vi "Loop_SOL.vi"() -> ()   [LabVIEW 2017, in "Wing.lvlib"]
uses:
  Wing.lvlib
  <vilib>/Rock Robotics/WPI/Solenoid/WPI_SolenoidValue.ctl
  <vilib>/Rock Robotics/WPI/Solenoid/WPI_SolenoidChannel.ctl
  <vilib>/Rock Robotics/WPI/Solenoid/WPI_SolenoidOpenSingle.vi
  _SHARE ALL/Global Share All/Global_STOP.vi
  Global_SM Write_Data Out.vi
  <vilib>/Rock Robotics/WPI/Solenoid/WPI_SolenoidSetEnum.vi
  <vilib>/Rock Robotics/WPI/Solenoid/WPI_SolenoidGetEnum.vi
  Global_ACT Write_Data Out.vi
panel:
  out "Value":T1
  out "Solenoid On.Off":bool
  out "Cycle Time (S)":dbl format="%.3g"
  in  "Target Time(ms)":u32=50
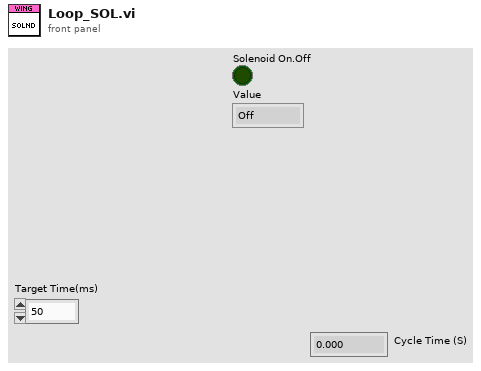
[diagram p1: front panel]
types:
  T1 = typedef "WPI_SolenoidValue.ctl" = enum16{"Off", "On", "Forward", "Reverse"}
  T2 = typedef "WPI_SolenoidChannel.ctl" = enum8{"Solenoid 0", "Solenoid 1", "Solenoid 2", "Solenoid 3", "Solenoid 4", "Solenoid 5", "Solenoid 6", "Solenoid 7", "Invalid"}
  T3 = typedef "WPI_SolenoidDevRef.ctl" = cluster{"DevStatus":errorcluster, "Pneumatics Control Module":u8, "Forward Solenoid Channel":T2, "Reverse Solenoid Channel":T2}
  T4 = cluster{"SolenoidDevRef":T3, "Target Time(ms)":u32, "Current Time":timestamp, "Previous Time":timestamp, "Cycle Time (S)":dbl, "Solenoid On.Off":bool, "Value":T1}
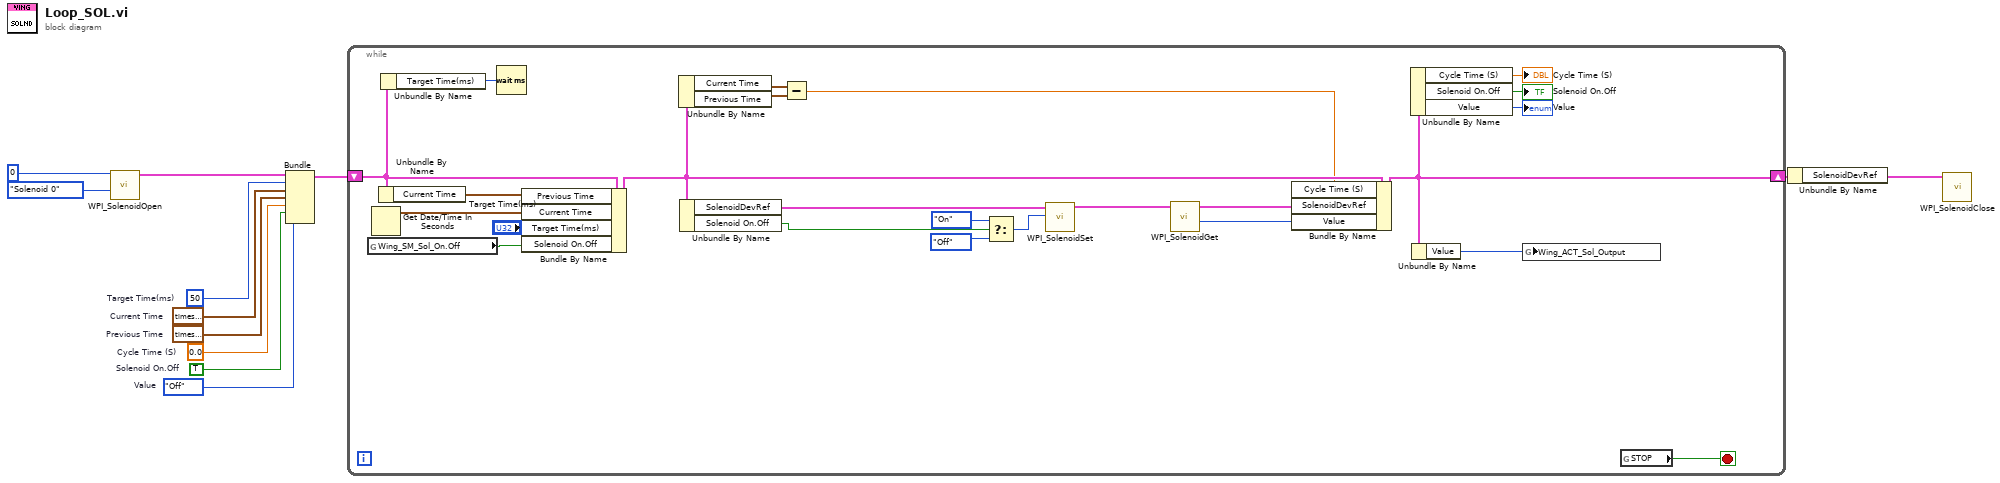
[diagram p0: block diagram]
diagram:
  w3 = WPI_SolenoidValue."Off"  # Value
  w4 = TRUE  # Solenoid On.Off
  w6 = 0.0  # Cycle Time (S)
  w12 = timestamp(0 s since 1904-01-01)  # Previous Time
  w11 = timestamp(0 s since 1904-01-01)  # Current Time
  w10 = u32 50  # Target Time(ms)
  n1 = call-poly <vilib>:"WPI_SolenoidOpen.vi"("Solenoid Channel"=WPI_SolenoidChannel."Solenoid 0", "Pneumatics Control Module (0)"=u8 0) -> ("SolenoidDevRef"=w5:T3)  [unwired: 8 in, 1 out]
  n2 = Bundle("SolenoidDevRef"=w5, "Target Time(ms)"=w10, "Current Time"=w11, "Previous Time"=w12, "Cycle Time (S)"=w6, "Solenoid On.Off"=w4, "Value"=w3) -> (w8:T4)  [unwired: 1 in]
  n3 = while {
    shift-right: [w26] -> w7
    shift-left: w8 -> [w28]
    stop <- w36 stop-if-true
    n4 = global read "Global_SM Write_Data Out.vi" "Wing_SM_Sol_On.Off"() -> (w22:bool)
    n5 = Get Date/Time In Seconds() -> (seconds since 1Jan1904=w34:timestamp)
    n6 = Unbundle By Name(w28) -> ("Current Time"=w33:timestamp)
    n7 = Unbundle By Name(w28) -> ("Target Time(ms)"=w27:u32)
    n8 = Wait (ms)(milliseconds to wait=w27) -> ()  [unwired: 1 out]
    n9 = Bundle By Name(cluster=w28, "Previous Time"=w33, "Current Time"=w34, "Target Time(ms)"="Target Time(ms)", "Solenoid On.Off"=w22) -> (w29:T4)
    n10 = Unbundle By Name(w29) -> ("Current Time"=w32:timestamp, "Previous Time"=w31:timestamp)
    n11 = Unbundle By Name(w29) -> ("SolenoidDevRef"=w35:T3, "Solenoid On.Off"=w21:bool)
    n12 = Subtract(x=w32, y=w31) -> (x-y=w24:dbl)
    n13 = Select(t=WPI_SolenoidValue."On" ("Value"), s=w21, f=WPI_SolenoidValue."Off" ("Value")) -> (s? t:f=w16:T1)
    n14 = call-poly <vilib>:"WPI_SolenoidSet.vi"("Value"=w16, "SolenoidDevRef"=w35) -> ("SolenoidDevRef"=w15:T3)  [unwired: 8 in, 1 out]
    n15 = call-poly <vilib>:"WPI_SolenoidGet.vi"("SolenoidDevRef"=w15) -> ("Value"=w20:T1, "SolenoidDevRef"=w23:T3)  [unwired: 8 in, 1 out]
    n16 = Bundle By Name(cluster=w29, "Cycle Time (S)"=w24, "SolenoidDevRef"=w23, "Value"=w20) -> (w26:T4)
    n17 = Unbundle By Name(w26) -> ("Cycle Time (S)"=→"Cycle Time (S)":dbl, "Solenoid On.Off"=→"Solenoid On.Off":bool, "Value"=→"Value":T1)
    n18 = Unbundle By Name(w26) -> ("Value"=w19:T1)
    n19 = global write "Global_ACT Write_Data Out.vi" "Wing_ACT_Sol_Output"(w19) -> ()
    n20 = global read "Global_STOP.vi" "STOP"() -> (w36:bool)
  }
  n21 = Unbundle By Name(w7) -> ("SolenoidDevRef"=w9:T3)
  n22 = call <vilib>:"WPI_SolenoidClose.vi"("SolenoidDevRef"=w9) -> ()  [unwired: 10 in, 1 out]
